vi "Main.vi"() -> ()   [LabVIEW 2018, in "Module Template.lvlib"]
uses:
  Module Template.lvlib
  Private/ctl/Message Data--cluster.ctl
  Private/ctl/State--enum.ctl
panel:
  in  "Shut other module":bool
  out "error out":errorcluster
  in  "Error in":errorcluster
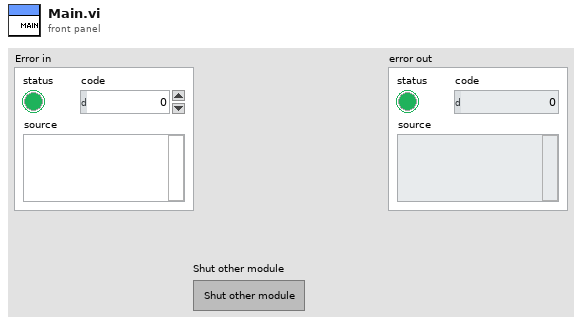
[diagram p1: front panel]
types:
  T1 = typedef "Module Template.lvlib/Message Data--cluster.ctl" = cluster{"State":T2, "Data":variant}
  T2 = typedef "Module Template.lvlib/State--enum.ctl" = enum16{"Initialize", "Error", "Shut Down", "Stop Module", "---", "Template", "Shut Module 2"}
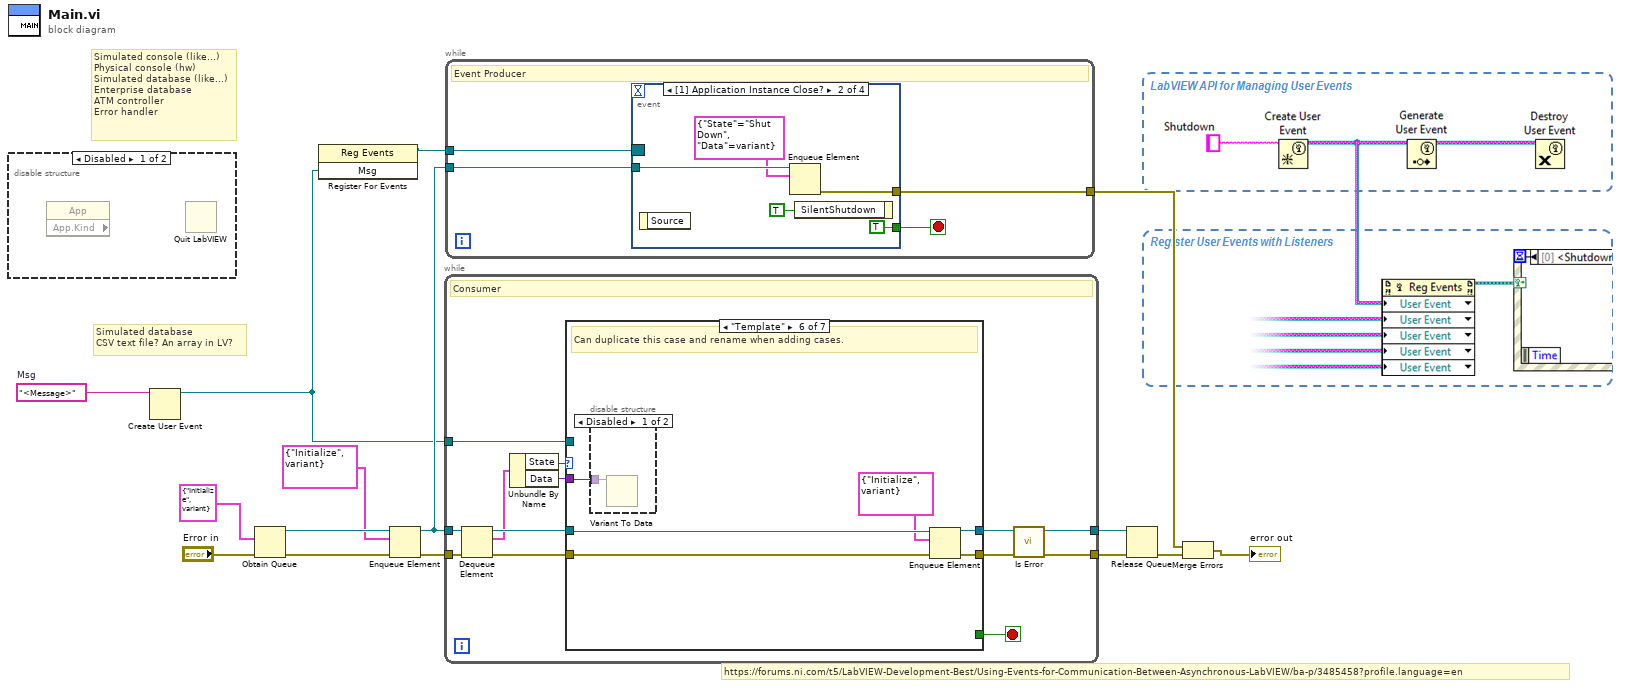
[diagram p0: block diagram]
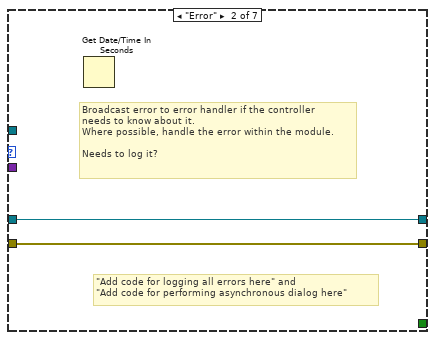
[diagram p4: hidden frame]
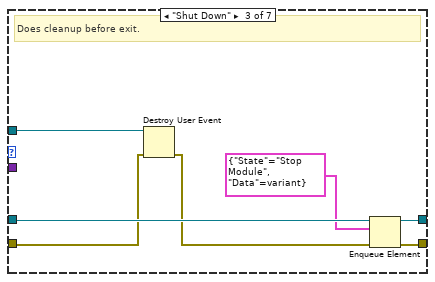
[diagram p5: hidden frame]
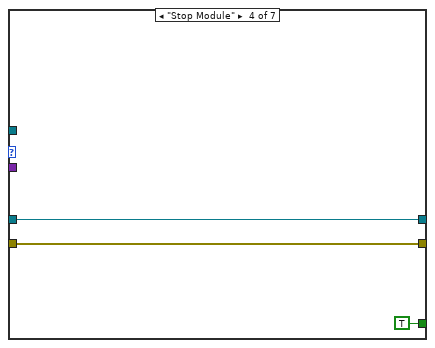
[diagram p6: hidden frame]
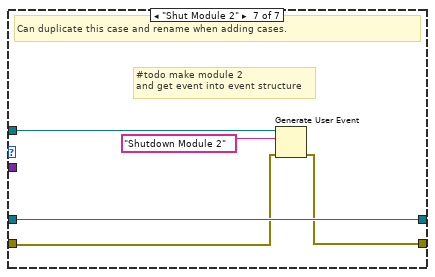
[diagram p9: hidden frame]
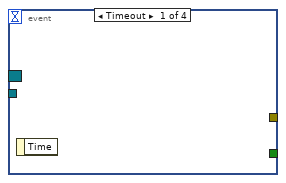
[diagram p10: hidden frame]
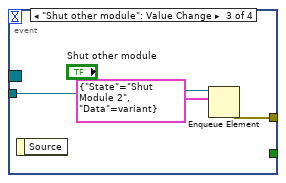
[diagram p11: hidden frame]
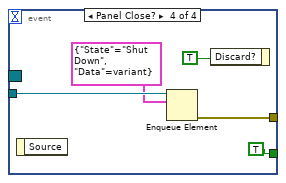
[diagram p12: hidden frame]
diagram:
  w3 = "<Message>"  # Msg
  # "https://forums.ni.com/t5/LabVIEW-Development-Best/Using-Events-for-Communication-Between-Asynchronous-LabVIEW/ba-p/3485458?profile.language=en"
  # "Simulated database\nCSV text file? An array in LV?"
  # "Simulated console (like...)\nPhysical console (hw)\nSimulated database (like...)\nEnterprise database \nATM controller\nError handler"
  n1 = disable-structure shown="Disabled" {
    frame Disabled {
      n2 = property class="App" props=["App.Kind"]() -> ()  [unwired: 2 in, 3 out]
      n3 = Quit LabVIEW() -> ()  [unwired: 1 in]
    }
    frame Enabled {
    }
  }
  n4 = Create User Event(user event datatype=w3) -> (user event=w1:refnum<user-event>)  [unwired: 1 in, 1 out]
  n5 = Obtain Queue(element data type=T1 {"State"=enum."Initialize", "Data"=variant} ("Message Data--cluster"), error in (no error)="Error in") -> (queue out=w10:refnum<queue>, error out=w15:errorcluster)  [unwired: 3 in, 1 out]
  n6 = register-events(w1) -> (reference out=w2:refnum<event-registration>)  [unwired: 2 in, 1 out]
  n7 = Enqueue Element(queue=w10, element=T1 {"State"=enum."Initialize", "Data"=variant}, error in (no error)=w15) -> (queue out=w9:refnum<queue>, error out=w14:errorcluster)  [unwired: 1 in, 1 out]
  n8 = while {
    tunnel: w9 -> [w28]
    tunnel: w14 -> [w27]
    tunnel: [w19] -> w12
    tunnel: [w20] -> w11
    tunnel: w1 -> [w16]
    stop <- w17 stop-if-true
    # "Consumer"
    n9 = Dequeue Element(queue=w28, error in (no error)=w27) -> (queue out=w26:refnum<queue>, element=w25:T1, error out=w23:errorcluster)  [unwired: 1 in, 1 out]
    n10 = Unbundle By Name(w25) -> ("State"=w24:T2, "Data"=w22:variant)
    n11 = case shown="\"Template\"" w24 {
      tunnel: w26 -> [w30 w32 w39 w41 w44 w47 w56]
      tunnel: [w30 w32 w38 w41 w44 w48 w56] -> w18
      tunnel: w23 -> [w29 w31 w34 w40 w43 w46 w53]
      tunnel: [w29 w31 w37 w40 w43 w49 w54] -> w21
      tunnel: w22 -> [_ _ _ _ _ w50 _]
      tunnel: [_ _ _ TRUE _ _ _] -> w17
      tunnel: w16 -> [_ _ w35 _ _ _ w52]
      frame "Initialize", Default {
      }
      frame "Error" {
        # "\"Add code for logging all errors here\" and \n\"Add code for performing asynchronous dialog here\""
        # "Broadcast error to error handler if the controller \nneeds to know about it.\nWhere possible, handle the error within the module.\n\nNeeds to log it?"
        n12 = Get Date/Time In Seconds() -> ()  [unwired: 1 out]
      }
      frame "Shut Down" {
        # "Does cleanup before exit."
        n13 = Destroy User Event(user event=w35, error in=w34) -> (error out=w33:errorcluster)
        n14 = Enqueue Element(queue=w39, element=T1 {"State"=enum."Stop Module", "Data"=variant}, error in (no error)=w33) -> (queue out=w38:refnum<queue>, error out=w37:errorcluster)  [unwired: 1 in, 1 out]
      }
      frame "Stop Module" {
      }
      frame "---" {
        # "Divider - no code."
      }
      frame "Template" {
        # "Can duplicate this case and rename when adding cases."
        n15 = disable-structure shown="Disabled" {
          disable-tunnel: w50 -> [w51 _]
          frame Disabled {
            n16 = Variant To Data(Variant=w51) -> ()  [unwired: 2 in, 2 out]
          }
          frame Enabled {
          }
        }
        n17 = Enqueue Element(queue=w47, element=T1 {"State"=enum."Initialize", "Data"=variant}, error in (no error)=w46) -> (queue out=w48:refnum<queue>, error out=w49:errorcluster)  [unwired: 1 in, 1 out]
      }
      frame "Shut Module 2" {
        # "#todo make module 2\nand get event into event structure"
        # "Can duplicate this case and rename when adding cases."
        n18 = Generate User Event(user event=w52, event data cluster="Shutdown Module 2" ("event data"), error in=w53) -> (error out=w54:errorcluster)  [unwired: 1 in, 1 out]
      }
    }
    n19 = call "Is Error.vi"("error in"=w21, "Queue in"=w18) -> ("error out"=w20:errorcluster, "Queue out"=w19:refnum<queue>)  [unwired: 8 in]
  }
  n20 = while {
    tunnel: w9 -> [w60]
    tunnel: [w59] -> w4
    tunnel: w2 -> [w57]
    stop <- w58 stop-if-true
    # "Event Producer"
    n21 = event shown="[1] Application Instance Close?" {
      selector: w57 -> [_ _ _ _]
      dyn-events: _ -> [_ _ _ _]
      timeout: _ -> [_ _ _ _]
      tunnel: w60 -> [_ w63 w68 w71]
      tunnel: [_ w64 w67 w72] -> w59
      tunnel: [_ TRUE _ TRUE] -> w58
      event Timeout {
        n22 = event-data() -> ()  [unwired: 1 in, 1 out]
      }
      event Application Instance Close? {
        n23 = event-data() -> ()  [unwired: 1 in, 1 out]
        n24 = Enqueue Element(queue=w63, element=T1 {"State"=enum."Shut Down", "Data"=variant}) -> (error out=w64:errorcluster)  [unwired: 2 in, 2 out]
        n25 = event-data("SilentShutdown"=TRUE) -> ()  [unwired: 1 in, 1 out]
      }
      event "Shut other module": Value Change {
        n26 = event-data() -> ()  [unwired: 1 in, 1 out]
        n27 = Enqueue Element(queue=w68, element=T1 {"State"=enum."Shut Module 2", "Data"=variant}) -> (error out=w67:errorcluster)  [unwired: 2 in, 2 out]
      }
      event Panel Close? {
        n28 = event-data() -> ()  [unwired: 1 in, 1 out]
        n29 = Enqueue Element(queue=w71, element=T1 {"State"=enum."Shut Down", "Data"=variant}) -> (error out=w72:errorcluster)  [unwired: 2 in, 2 out]
        n30 = event-data("Discard?"=TRUE ("SilentShutdown")) -> ()  [unwired: 1 in, 1 out]
      }
    }
  }
  n31 = Release Queue(queue=w12, error in (no error)=w11) -> (error out=w5:errorcluster)  [unwired: 1 in, 2 out]
  n32 = Merge Errors(w4, w5) -> (→"error out":errorcluster)
